vi "Read TemplatesFolder Key (create if does not exist).vi"(8 "Error In":errorcluster) -> (0 "Error Out":errorcluster)   [LabVIEW 2021]
doc: "<add documentation here>"
uses:
  <vilib>/registry/registry.llb/Write Registry Value Simple STR.vi
panel:
  out "Templates Folder Path":string
  # "Development\nControls or indicators that are useful for development or testing, but which are not outputs of the VI."
  # "Input\nInputs to the VI"
  # "Output\nOutputs of the VI"
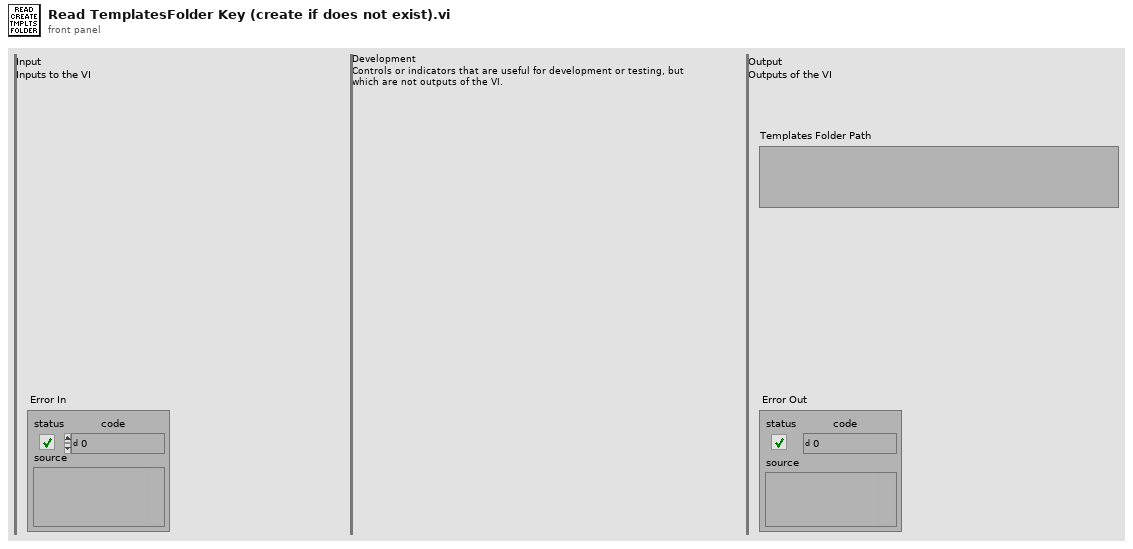
[diagram p1: front panel]
types:
  T1 = enum32{"Unknown", "REG_CREATED_NEW_KEY", "REG_OPENED_EXISTING_KEY"}
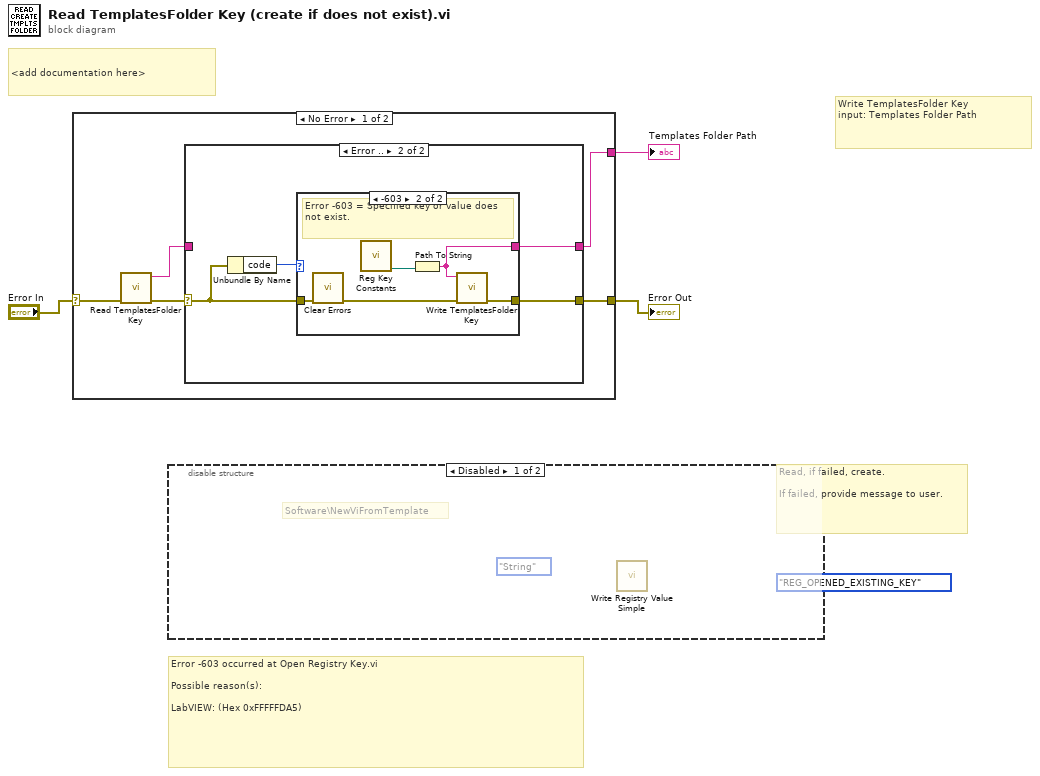
[diagram p0: block diagram]
diagram:
  (unwired) T1."REG_OPENED_EXISTING_KEY" ("action taken")
  # "Write TemplatesFolder Key\ninput: Templates Folder Path"
  # "Read, if failed, create.\n\nIf failed, provide message to user."
  # "Error -603 occurred at Open Registry Key.vi\n\nPossible reason(s):\n\nLabVIEW: (Hex 0xFFFFFDA5)"
  # "<add documentation here>"
  n1 = case shown="No Error" "Error In" {
    selector: "Error In" -> [w8 w21]
    tunnel: [w6 w21] -> w2
    tunnel: [w5 _] -> w1
    frame No Error {
      n2 = call "Read TemplatesFolder Key.vi"("Error In"=w8) -> ("Error Out"=w7:errorcluster, "Templates Folder Path"=w4:string)  [unwired: 9 in]
      n3 = case shown="Error .." w7 {
        selector: w7 -> [w10 w12]
        tunnel: [w10 w14] -> w6
        tunnel: [w9 w13] -> w5
        tunnel: w4 -> [w9 _]
        frame No Error {
        }
        frame Error {
          n4 = Unbundle By Name(w12) -> ("code"=w11:i32)
          n5 = case shown="-603" w11 {
            tunnel: w12 -> [w15 w20]
            tunnel: [w15 w18] -> w14
            tunnel: [_ w16] -> w13
            frame Default {
            }
            frame -603 {
              # "Error -603 = Specified key or value does not exist."
              n6 = call <vilib>:"Clear Errors.vi"("error in (no error)"=w20) -> ("error out"=w19:errorcluster)  [unwired: 5 in, 1 out]
              n7 = call "Reg Key Constants.vi"() -> ("Default Templates Folder"=w17:path)  [unwired: 4 in, 3 out]
              n8 = Path To String(path=w17) -> (string=w16:string)
              n9 = call "Write TemplatesFolder Key.vi"("Error In"=w19, "Templates Folder Path"=w16) -> ("Error Out"=w18:errorcluster)  [unwired: 9 in]
            }
          }
        }
      }
    }
    frame Error {
    }
  }
  "Error Out" <- w2
  "Templates Folder Path" <- w1
  n10 = disable-structure shown="Disabled" {
    frame Disabled {
      (unwired) enum16{"String", "Binary", "DWORD"}."String" ("simple data type")
      # "Software\\NewViFromTemplate"
      n11 = call-poly <vilib>:"Write Registry Value Simple.vi"() -> ()  [unwired: 8 in, 2 out]
    }
    frame Enabled {
    }
  }
